vi "Osc Control.vi"(0 "RedPitaya connection in":refnum<k5>, 2 "Command":string(combo)="RST", 5 "error in":errorcluster, 12 "timeout ms (2000)":i32=2000) -> (14 "RedPitaya connection out":refnum<k5>, 19 "error out":errorcluster)   [LabVIEW 2010, in "RedPitaya.lvlib"]
doc: "Executes commands on oscilloscope.\nPossible commands: reset, stop, run, single, autoscale"
uses:
  RedPitaya.lvlib
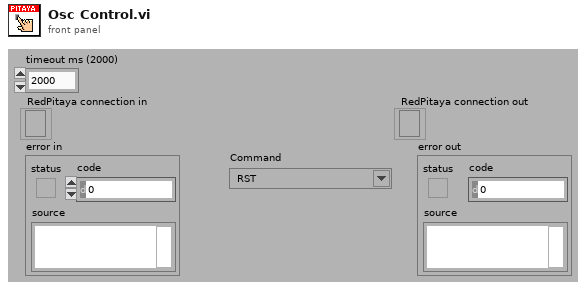
[diagram p1: front panel]
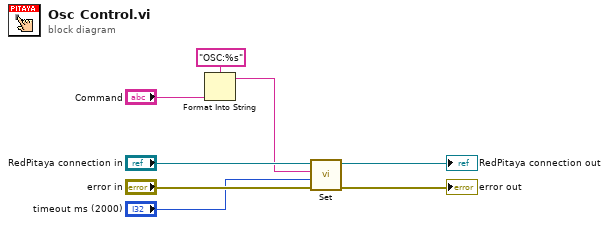
[diagram p0: block diagram]
diagram:
  n1 = Format Into String(format string="OSC:%s", "Command") -> (resulting string=w2:string)  [unwired: 2 in, 1 out]
  n2 = call "Set.vi"("error in"="error in", "timeout ms (2000)"="timeout ms (2000)", "SCPI Message"=w2, "RedPitaya connection in"="RedPitaya connection in") -> ("error out"=→"error out":errorcluster, "RedPitaya connection out"=→"RedPitaya connection out":refnum<k5>)  [unwired: 5 in, 1 out]
